vi "ABCtoAlphaBeta_3PhasePowInv.vi"(0 "A":sgl, 5 "B":sgl, 7 "C":sgl, 12 "Resources":T1) -> (4 "alpha":sgl, 6 "beta":sgl)   [LabVIEW 2017]
uses:
  Multiplier/Multiplier.lvclass
  Adder/Adder.lvclass
  Subtractor/Subtractor.lvclass
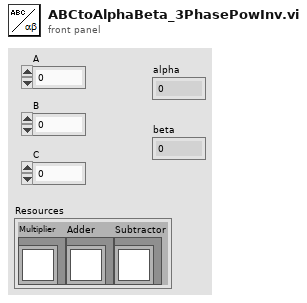
[diagram p1: front panel]
types:
  T1 = cluster{"Multiplier":refnum<class "Multiplier.lvclass">, "Adder":refnum<class "Adder.lvclass">, "Subtractor":refnum<class "Subtractor.lvclass">}
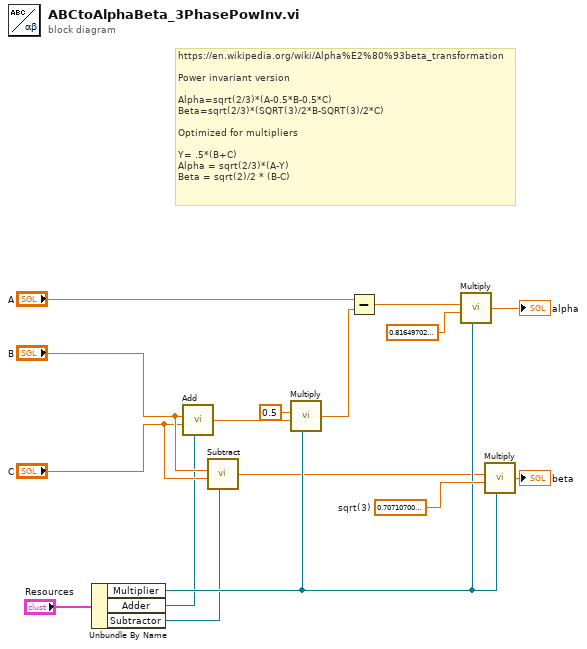
[diagram p0: block diagram]
diagram:
  w15 = sgl 0.707107  # sqrt(3)
  # "https://en.wikipedia.org/wiki/Alpha%E2%80%93beta_transformation\n\nPower invariant version\n\nAlpha=sqrt(2/3)*(A-0.5*B-0.5*C)\nBeta=sqrt(2/3)*(SQRT(3)/2*B-SQRT(3)/2*C)\n\nOptimized for multipliers\n\nY= .5*(B+C)\nAlpha = sqrt(2/3)*(A-Y)\nBeta = sqrt(2)/2 * (B-C)"
  n1 = Unbundle By Name("Resources") -> ("Multiplier"=w7:refnum<class "Multiplier.lvclass">, "Adder"=w1:refnum<class "Adder.lvclass">, "Subtractor"=w5:refnum<class "Subtractor.lvclass">)
  n2 = call-dynamic "Add.vi"("x"="B", "y"="C", "Adder"=w1) -> ("x+y"=w4:sgl)  [unwired: 4 in]
  n3 = call-dynamic "Subtract.vi"("x"="B", "y"="C", "Subtractor"=w5) -> ("x-y"=w6:sgl)  [unwired: 4 in]
  n4 = call-dynamic "Multiply.vi"("x"=sgl 0.5, "y"=w4, "Multiplier"=w7) -> ("x*y"=w10:sgl)  [unwired: 4 in]
  n5 = Subtract(x="A", y=w10) -> (x-y=w13:sgl)
  n6 = call-dynamic "Multiply.vi"("x"=w13, "y"=sgl 0.816497, "Multiplier"=w7) -> ("x*y"=→"alpha":sgl)  [unwired: 4 in]
  n7 = call-dynamic "Multiply.vi"("x"=w6, "y"=w15, "Multiplier"=w7) -> ("x*y"=→"beta":sgl)  [unwired: 4 in]
